vi "PH_Beamline_Chief.set States in GUI.vi"(0 "i ref in":refnum<vi>, 5 "error in":errorcluster) -> (14 "i ref out":refnum<vi>, 19 "error out":errorcluster)   [LabVIEW 2014]
uses:
  PH_BL-Master/PH_BL-Master.lvlib
  PH_Beamline_Chief.lvlib
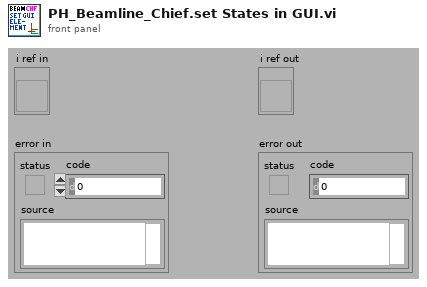
[diagram p1: front panel]
types:
  T1 = typedef "PH_BL-Master.lvlib/PH_BL-Master.i attribute.ctl" = cluster{"GUI Refs":cluster{"Delete":refnum<vi>}, "Remote Controlled by":string, "Boolean Condition Service Subscriber":refnum<vi>[], "Picture Condition Service Subscriber":refnum<vi>[], "R2S":cluster{"GUI Ref":refnum<vi>, "State":bool}, "Vacua":cluster{"GUI Ref":refnum<vi>, "Limit":dbl, "Curr Value":dbl, "in range":bool}[], "O2 Inspection":cluster{"GUI Ref":refnum<vi>, "Concentration":dbl, "State":T2}[], "Boolean Status Service Subscriber":cluster{"GUI Ref":refnum<vi>, "Status":T2, "no Link?":bool, "Status Subscriber Class":T3}[], "Picture Status Service Subscriber":cluster{"GUI Ref":refnum<vi>, "Status":T2, "no Link?":bool, "Status Subscriber Class":T3}[], "6P 4Q Service Subscriber":cluster{"GUI Ref":refnum<vi>, "Selector":T4, "no Link?":bool}[], "Index of latest 6P 4Q changing Instance":i32, "Index of latest Picture Status changing Instance":i32, "Index of latest Boolean Status changing Instance":i32, "Vision ID on same Node":string, "Start Phase over?":bool}
  T2 = typedef "Status.ctl" = i16
  T3 = typedef "PH_BL-Master.lvlib/PH_BL-Master.Status Subscriber Class.ctl" = enum16{"unknown", "Switch", "BB", "6P Switch", "Switch GUI", "Switch and 6P State"}
  T4 = typedef "PH_4_Pos_Selector.lvlib/PH_4_Pos_Selector.Position Selector.ctl" = u16
  T5 = cluster{"GUI Ref":refnum<vi>, "Status":T2, "no Link?":bool, "Status Subscriber Class":T3}[]
  T6 = cluster{"GUI Ref":refnum<vi>, "Status":T2, "no Link?":bool, "Status Subscriber Class":T3}
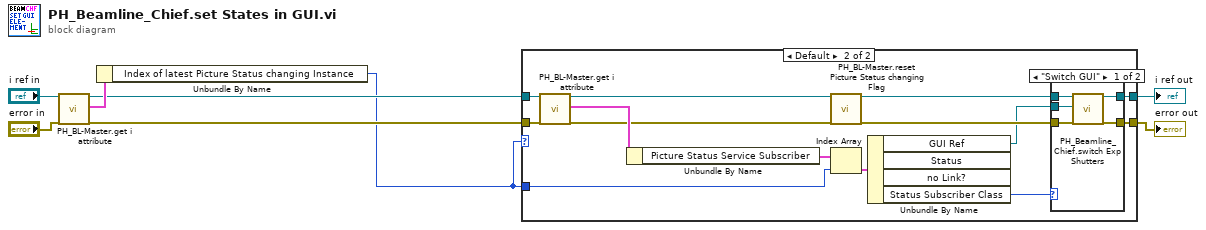
[diagram p0: block diagram]
diagram:
  n1 = call "PH_BL-Master.get i attribute.vi"("i ref in"="i ref in", "error in (no error)"="error in") -> ("i ref out"=w4:refnum<vi>, "i attribute"=w8:T1, "error out"=w5:errorcluster)  [unwired: 15 in]
  n2 = Unbundle By Name(w8) -> ("Index of latest Picture Status changing Instance"=w1:i32)
  n3 = case shown="Default" w1 {
    tunnel: [w10 w20] -> w3
    tunnel: [w9 w19] -> w2
    tunnel: w5 -> [w9 w24]
    tunnel: w4 -> [w10 w23]
    tunnel: w1 -> [_ w13]
    frame -1 {
    }
    frame Default {
      n4 = call "PH_BL-Master.get i attribute.vi"("i ref in"=w23, "error in (no error)"=w24) -> ("i ref out"=w16:refnum<vi>, "i attribute"=w22:T1, "error out"=w18:errorcluster)  [unwired: 15 in]
      n5 = Unbundle By Name(w22) -> ("Picture Status Service Subscriber"=w12:T5)
      n6 = call "PH_BL-Master.reset Picture Status changing Flag.vi"("i ref in"=w16, "error in"=w18) -> ("i ref out"=w15:refnum<vi>, "error out"=w17:errorcluster)  [unwired: 16 in]
      n7 = Index Array(array=w12, index=w13) -> (element=w11:T6)
      n8 = Unbundle By Name(w11) -> ("GUI Ref"=w14:refnum<vi>, "Status Subscriber Class"=w21:T3)  [unwired: 2 out]
      n9 = case shown="\"Switch GUI\"" w21 {
        tunnel: [w29 w31] -> w20
        tunnel: [w28 w30] -> w19
        tunnel: w17 -> [w27 w30]
        tunnel: w15 -> [w26 w31]
        tunnel: w14 -> [w25 _]
        frame "Switch GUI" {
          n10 = call "PH_Beamline_Chief.switch Exp Shutters.vi"("i ref in"=w26, 2:w25, "error in"=w27) -> ("i ref out"=w29:refnum<vi>, "error out"=w28:errorcluster)  [unwired: 15 in]
        }
        frame Default {
        }
      }
    }
  }
  "error out" <- w2
  "i ref out" <- w3
